vi "Bezier.vi"(2 "Segments":dbl, 3 "Parameters":cluster{"X":dbl, "Y":dbl}[](array[cluster])) -> (0 "XY Graph":cluster{dbl[], dbl[]}[](array[cluster]), 1 "Coordinate Array":cluster{"X":dbl, "Y":dbl}[](array[cluster]))   [LabVIEW 2019]
doc: "This VI uses the equation for a Bézier curve to create a set of coordinates."
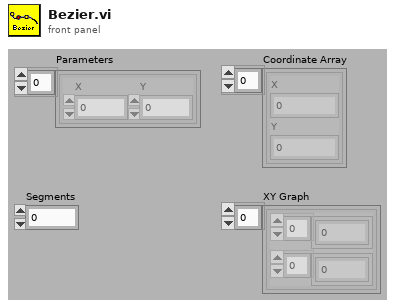
[diagram p1: front panel]
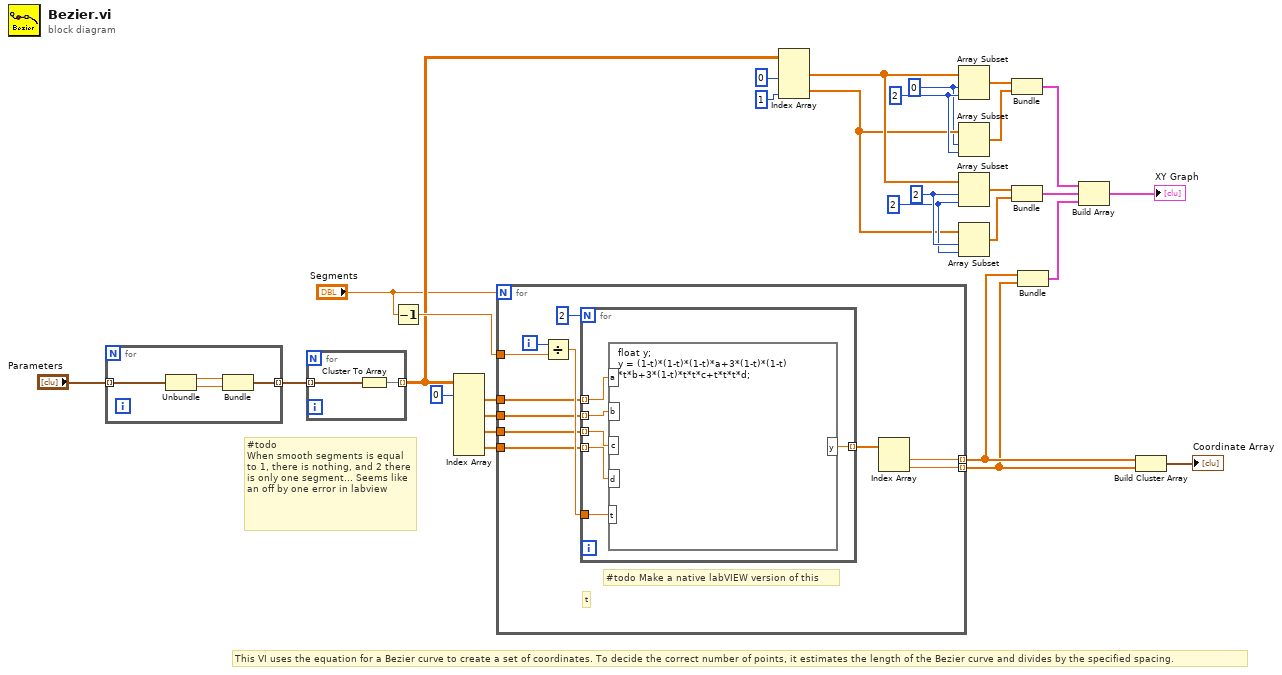
[diagram p0: block diagram]
diagram:
  w25 = 2 ("length")
  w26 = 2 ("index")
  w27 = 2 ("length")
  w1 = 0 ("index")
  # "#todo\nWhen smooth segments is equal to 1, there is nothing, and 2 there is only one segment... Seems like an off by one error in labview"
  # "This VI uses the equation for a Bezier curve to create a set of coordinates. To decide the correct number of points, it estimates the length of the Bezier curve and divides by the specified spacing."
  n1 = for {
    tunnel: "Parameters" -> [w33] mode=indexing
    tunnel: [w31] -> w5 mode=indexing
    n2 = Unbundle(w33) -> ("X"=w32:dbl, "Y"=w30:dbl)
    n3 = Bundle("X"=w32, "Y"=w30) -> (w31:cluster{"X":dbl, "Y":dbl})  [unwired: 1 in]
  }
  n4 = for {
    tunnel: w5 -> [w35] mode=indexing
    tunnel: [w34] -> w7 mode=indexing
    n5 = Cluster To Array(cluster=w35) -> (array=w34:dbl[])
  }
  n6 = Decrement(x="Segments") -> (x-1=w15:dbl)
  n7 = Index Array(array=w7, index (row) #1=0 ("index (row)")) -> (element #1=w13:dbl[], element #2=w12:dbl[], element #3=w11:dbl[], element #4=w10:dbl[])  [unwired: 7 in]
  n8 = for {
    N: "Segments" -> [_]
    tunnel: w13 -> [w43]
    tunnel: w15 -> [w45]
    tunnel: w12 -> [w42]
    tunnel: w11 -> [w41]
    tunnel: w10 -> [w40]
    tunnel: [w38] -> w9 mode=indexing
    tunnel: [w37] -> w4 mode=indexing
    i -> [w46]
    # "#todo Make a native labVIEW version of this"
    # "t"
    n9 = Divide(x=w46, y=w45) -> (x/y=w44:dbl)
    n10 = for {
      N: 2 -> [_]
      tunnel: w44 -> [w52]
      tunnel: w43 -> [w51] mode=indexing
      tunnel: w42 -> [w50] mode=indexing
      tunnel: w41 -> [w49] mode=indexing
      tunnel: w40 -> [w48] mode=indexing
      tunnel: [w47] -> w39 mode=indexing
      n11 = formula code="float y;\ny = (1-t)*(1-t)*(1-t)*a+3*(1-t)*(1-t)\n*t*b+3*(1-t)*t*t*c+t*t*t*d;"("t"=w52, "a"=w51, "b"=w50, "c"=w49, "d"=w48) -> ("y"=w47:dbl)
    }
    n12 = Index Array(array=w39) -> (element #1=w38:dbl, element #2=w37:dbl)  [unwired: 2 in]
  }
  n13 = Index Array(array=w7, index (col) #1=0 ("disabled index (col)"), index (col) #2=1 ("index (col)")) -> (element #1=w24:dbl[], element #2=w2:dbl[])  [unwired: 2 in]
  n14 = Array Subset(array=w24, index=w1, length=w27) -> (w20:dbl[])
  n15 = Array Subset(array=w2, index=w1, length=w27) -> (w19:dbl[])
  n16 = Array Subset(array=w24, index=w26, length=w25) -> (w18:dbl[])
  n17 = Array Subset(array=w2, index=w26, length=w25) -> (w17:dbl[])
  n18 = Bundle(w20, w19) -> (w23:cluster{dbl[], dbl[]})  [unwired: 1 in]
  n19 = Bundle(w18, w17) -> (w22:cluster{dbl[], dbl[]})  [unwired: 1 in]
  n20 = Bundle(w9, w4) -> (w16:cluster{dbl[], dbl[]})  [unwired: 1 in]
  n21 = Build Array(w23, w22, w16) -> (→"XY Graph":cluster{dbl[], dbl[]}[])
  n22 = Build Cluster Array(w9, w4) -> (→"Coordinate Array":cluster{dbl, dbl}[])
